vi "Get_Set_Alignment_Parameters.vi"(6 "Get/Set":T2, 8 "Status/Errors in":refnum<vi>, 9 "Alignment parameters in":refnum<vi>, 10 "Value in":T1 {"SLV Ch. 2"."Gain adjust neg." format="%02x"; "SLV Ch. 2"."Gain adjust pos." format="%02x"; "SLV Ch. 2"."Offset adjust neg." format="%02x"; "SLV Ch. 2"."Offset adjust pos." format="%02x"; "SLV Ch. 1"."Gain adjust neg." format="%02x"; "SLV Ch. 1"."Gain adjust pos." format="%02x"; "SLV Ch. 1"."Offset adjust neg." format="%02x"; "SLV Ch. 1"."Offset adjust pos." format="%02x"; "MAS Ch. 2"."Gain adjust neg." format="%02x"; "MAS Ch. 2"."Gain adjust pos." format="%02x"; "MAS Ch. 2"."Offset adjust neg." format="%02x"; "MAS Ch. 2"."Offset adjust pos." format="%02x"; "Full scale SLV" format="%02x"; "Comm. offset SLV" format="%02x"; "Coinc. time" format="%04x"; "Pre coinc. time" format="%04x"; "Post coinc. time" format="%04x"; "MAS Ch. 1"."Gain adjust neg." format="%02x"; "MAS Ch. 1"."Gain adjust pos." format="%02x"; "MAS Ch. 1"."Offset adjust neg." format="%02x"; "MAS Ch. 1"."Offset adjust pos." format="%02x"; "Full scale MAS" format="%02x"; "Comm. offset MAS" format="%02x"; "Trigger condition" format="%02x"}) -> (0 "Status/Errors out":refnum<vi>, 1 "Alignment parameters out":refnum<vi>, 2 "Value out":T1 {"SLV Ch. 2"."Gain adjust neg." format="%02x"; "SLV Ch. 2"."Gain adjust pos." format="%02x"; "SLV Ch. 2"."Offset adjust neg." format="%02x"; "SLV Ch. 2"."Offset adjust pos." format="%02x"; "SLV Ch. 1"."Gain adjust neg." format="%02x"; "SLV Ch. 1"."Gain adjust pos." format="%02x"; "SLV Ch. 1"."Offset adjust neg." format="%02x"; "SLV Ch. 1"."Offset adjust pos." format="%02x"; "MAS Ch. 2"."Gain adjust neg." format="%02x"; "MAS Ch. 2"."Gain adjust pos." format="%02x"; "MAS Ch. 2"."Offset adjust neg." format="%02x"; "MAS Ch. 2"."Offset adjust pos." format="%02x"; "Full scale SLV" format="%02x"; "Comm. offset SLV" format="%02x"; "Coinc. time" format="%04x"; "Pre coinc. time" format="%04x"; "Post coinc. time" format="%04x"; "MAS Ch. 1"."Gain adjust neg." format="%02x"; "MAS Ch. 1"."Gain adjust pos." format="%02x"; "MAS Ch. 1"."Offset adjust neg." format="%02x"; "MAS Ch. 1"."Offset adjust pos." format="%02x"; "Full scale MAS" format="%02x"; "Comm. offset MAS" format="%02x"; "Trigger condition" format="%02x"})   [LabVIEW 2013]
uses:
  Controls/Get_Set_Calibration_Options.ctl
  Controls/Calibration_Parameters.ctl
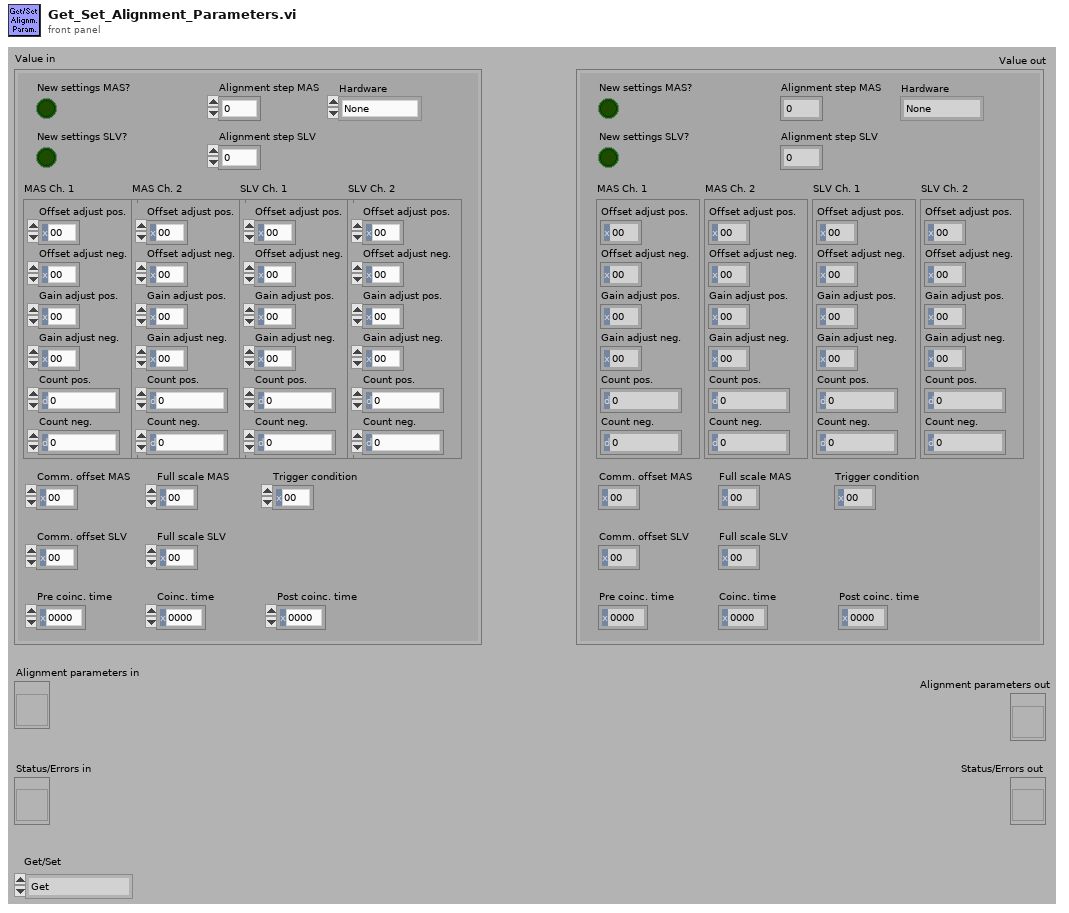
[diagram p1: front panel]
types:
  T1 = typedef "Calibration_Parameters.ctl" = cluster{"New settings MAS?":bool, "New settings SLV?":bool, "Alignment step MAS":i32, "Alignment step SLV":i32, "MAS Ch. 1":cluster{"Offset adjust pos.":u8, "Offset adjust neg.":u8, "Gain adjust pos.":u8, "Gain adjust neg.":u8, "Count pos.":dbl, "Count neg.":dbl}, "MAS Ch. 2":cluster{"Offset adjust pos.":u8, "Offset adjust neg.":u8, "Gain adjust pos.":u8, "Gain adjust neg.":u8, "Count pos.":dbl, "Count neg.":dbl}, "SLV Ch. 1":cluster{"Offset adjust pos.":u8, "Offset adjust neg.":u8, "Gain adjust pos.":u8, "Gain adjust neg.":u8, "Count pos.":dbl, "Count neg.":dbl}, "SLV Ch. 2":cluster{"Offset adjust pos.":u8, "Offset adjust neg.":u8, "Gain adjust pos.":u8, "Gain adjust neg.":u8, "Count pos.":dbl, "Count neg.":dbl}, "Comm. offset MAS":u8, "Full scale MAS":u8, "Comm. offset SLV":u8, "Full scale SLV":u8, "Trigger condition":u8, "Pre coinc. time":u16, "Coinc. time":u16, "Post coinc. time":u16, "Hardware":enum8{"None", "HiSPARC I", "HiSPARC II", "HiSPARC III", "Unknown"}}
  T2 = typedef "Get_Set_Calibration_Options.ctl" = enum16{"Get", "Set", "Set MAS", "Set SLV"}
  T3 = cluster{"New settings MAS?":bool, "New settings SLV?":bool, "Alignment step MAS":i32, "Alignment step SLV":i32, "MAS Ch. 1":cluster{"Offset adjust pos.":u8, "Offset adjust neg.":u8, "Gain adjust pos.":u8, "Gain adjust neg.":u8, "Count pos.":dbl, "Count neg.":dbl}, "MAS Ch. 2":cluster{"Offset adjust pos.":u8, "Offset adjust neg.":u8, "Gain adjust pos.":u8, "Gain adjust neg.":u8, "Count pos.":dbl, "Count neg.":dbl}, "SLV Ch. 1":cluster{"Offset adjust pos.":u8, "Offset adjust neg.":u8, "Gain adjust pos.":u8, "Gain adjust neg.":u8, "Count pos.":dbl, "Count neg.":dbl}, "SLV Ch. 2":cluster{"Offset adjust pos.":u8, "Offset adjust neg.":u8, "Gain adjust pos.":u8, "Gain adjust neg.":u8, "Count pos.":dbl, "Count neg.":dbl}, "Comm. offset MAS":u8, "Full scale MAS":u8, "Comm. offset SLV":u8, "Full scale SLV":u8, "Trigger condition":u8, "Pre coinc. time":u16, "Coinc. time":u16, "Post coinc. time":u16, "Hardware":enum8{"None", "HiSPARC I", "HiSPARC II", "HiSPARC III", "Unknown"}}
  T4 = cluster{"Offset adjust pos.":u8, "Offset adjust neg.":u8, "Gain adjust pos.":u8, "Gain adjust neg.":u8, "Count pos.":dbl, "Count neg.":dbl}
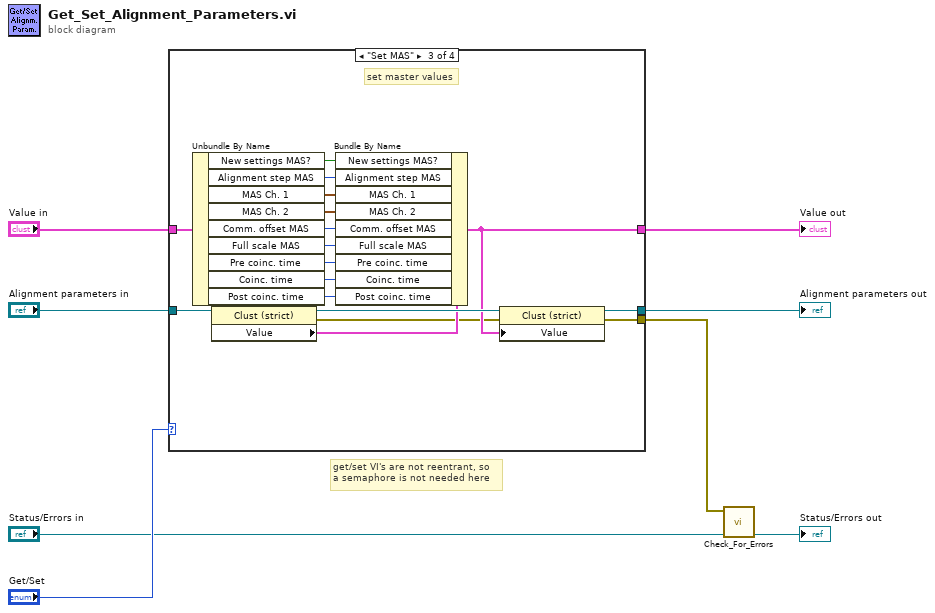
[diagram p0: block diagram]
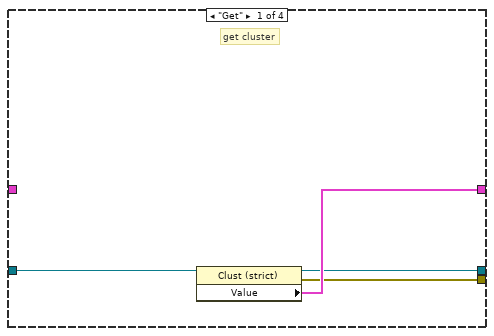
[diagram p2: hidden frame]
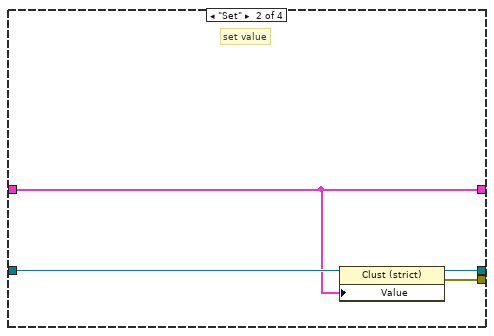
[diagram p3: hidden frame]
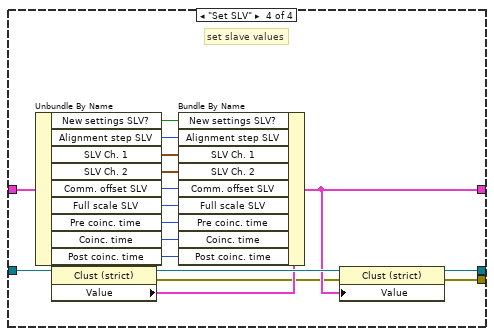
[diagram p4: hidden frame]
diagram:
  # "get/set VI's are not reentrant, so\na semaphore is not needed here"
  n1 = case shown="\"Set MAS\"" "Get/Set" {
    tunnel: "Value in" -> [_ w13 w31 w48]
    tunnel: "Alignment parameters in" -> [w12 w16 w30 w47]
    tunnel: [w9 w15 w33 w50] -> w1
    tunnel: [w10 w14 w32 w49] -> w6
    tunnel: [w11 w13 w27 w44] -> w3
    frame "Get" {
      # "get cluster"
      n2 = property class="Clust (strict)"(reference=w12) -> (reference out=w9:refnum<vi>, error out=w10:errorcluster, "Value"=w11:T3)  [unwired: 1 in]
    }
    frame "Set" {
      # "set value"
      n3 = property class="Clust (strict)"(reference=w16, "Value"=w13) -> (reference out=w15:refnum<vi>, error out=w14:errorcluster)  [unwired: 1 in]
    }
    frame "Set MAS" {
      # "set master values"
      n4 = Unbundle By Name(w31) -> ("New settings MAS?"=w26:bool, "Alignment step MAS"=w25:i32, "MAS Ch. 1"=w24:T4, "MAS Ch. 2"=w23:T4, "Comm. offset MAS"=w22:u8, "Full scale MAS"=w21:u8, "Pre coinc. time"=w19:u16, "Coinc. time"=w18:u16, "Post coinc. time"=w17:u16)
      n5 = property class="Clust (strict)"(reference=w30) -> (reference out=w29:refnum<vi>, error out=w20:errorcluster, "Value"=w28:T3)  [unwired: 1 in]
      n6 = Bundle By Name(cluster=w28, "New settings MAS?"=w26, "Alignment step MAS"=w25, "MAS Ch. 1"=w24, "MAS Ch. 2"=w23, "Comm. offset MAS"=w22, "Full scale MAS"=w21, "Pre coinc. time"=w19, "Coinc. time"=w18, "Post coinc. time"=w17) -> (w27:T3)
      n7 = property class="Clust (strict)"(reference=w29, error in=w20, "Value"=w27) -> (reference out=w33:refnum<vi>, error out=w32:errorcluster)
    }
    frame "Set SLV" {
      # "set slave values"
      n8 = Unbundle By Name(w48) -> ("New settings SLV?"=w43:bool, "Alignment step SLV"=w42:i32, "SLV Ch. 1"=w41:T4, "SLV Ch. 2"=w40:T4, "Comm. offset SLV"=w39:u8, "Full scale SLV"=w38:u8, "Pre coinc. time"=w36:u16, "Coinc. time"=w35:u16, "Post coinc. time"=w34:u16)
      n9 = property class="Clust (strict)"(reference=w47) -> (reference out=w46:refnum<vi>, error out=w37:errorcluster, "Value"=w45:T3)  [unwired: 1 in]
      n10 = Bundle By Name(cluster=w45, "New settings SLV?"=w43, "Alignment step SLV"=w42, "SLV Ch. 1"=w41, "SLV Ch. 2"=w40, "Comm. offset SLV"=w39, "Full scale SLV"=w38, "Pre coinc. time"=w36, "Coinc. time"=w35, "Post coinc. time"=w34) -> (w44:T3)
      n11 = property class="Clust (strict)"(reference=w46, error in=w37, "Value"=w44) -> (reference out=w50:refnum<vi>, error out=w49:errorcluster)
    }
  }
  "Value out" <- w3
  "Alignment parameters out" <- w1
  n12 = call "Check_For_Errors.vi"("Status/Errors in"="Status/Errors in", "error in"=w6) -> ("Status/Errors out"=→"Status/Errors out":refnum<vi>)  [unwired: 9 out]
